vi "Solve General Linear Equations with SVD (CDB).vi"(8 "iteration":i32=2, 9 "relative tolerance":dbl, 10 "Known Vector":cdb[](array[numeric]), 11 "Input Matrix":T1) -> (0 "error":i32, 3 "Solution Vector":cdb[](array[numeric]))   [LabVIEW 2020, in "NI_AALPro.lvlib"]
uses:
  NI_AALPro.lvlib
  ComplexMatrix.ctl
  NI_AALBase.lvlib
  NI_Matrix.lvlib
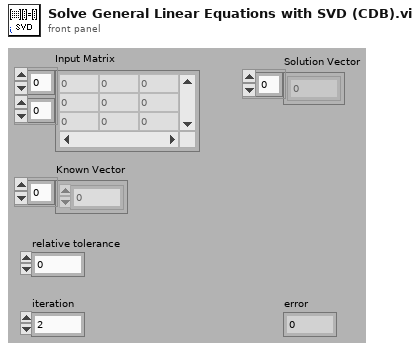
[diagram p1: front panel]
types:
  T1 = typedef "NI_Matrix.lvlib/ComplexMatrix.ctl" = cdb[][]
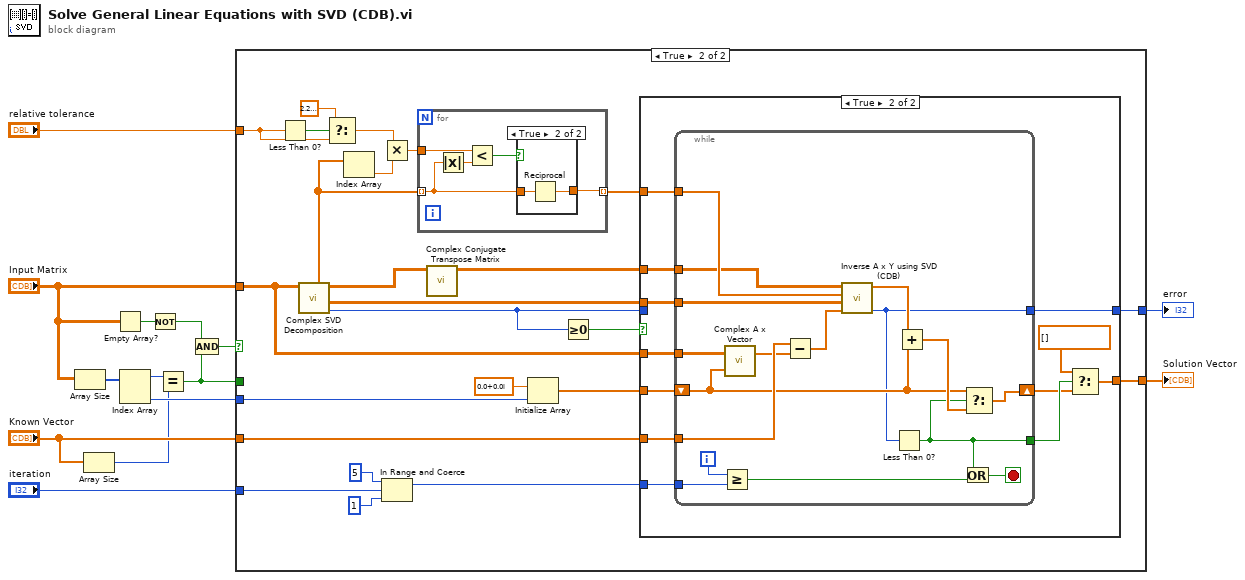
[diagram p0: block diagram]
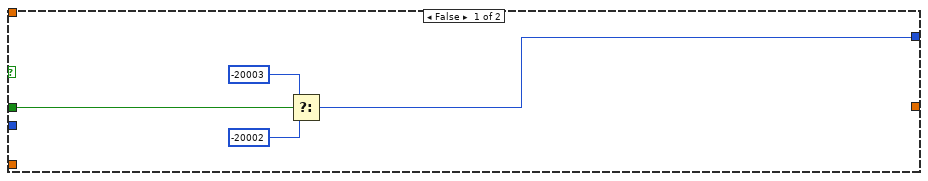
[diagram p2: hidden frame]
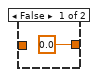
[diagram p4: hidden frame]
diagram:
  n1 = Array Size(array="Input Matrix") -> (size(s)=w12:i32[])
  n2 = Array Size(array="Known Vector") -> (size(s)=w6:i32)
  n3 = Empty Array?(array="Input Matrix") -> (empty?=w4:bool)
  n4 = Index Array(array=w12) -> (element #1=w7:i32, element #2=w9:i32)  [unwired: 2 in]
  n5 = Not(x=w4) -> (.not. x?=w3:bool)
  n6 = Equal?(x=w7, y=w6) -> (x = y?=w1:bool)
  n7 = Compound Arithmetic op=AND(w3, w1) -> (w2:bool)
  n8 = case shown="True" w2 {
    tunnel: "relative tolerance" -> [_ w41]
    tunnel: "iteration" -> [_ w31]
    tunnel: "Input Matrix" -> [_ w19]
    tunnel: [_ w24] -> w11
    tunnel: [w15 w23] -> w10
    tunnel: w9 -> [_ w21]
    tunnel: "Known Vector" -> [_ w20]
    tunnel: w1 -> [w18 _]
    frame False {
      n9 = Select(t=-20003 ("error"), s=w18, f=-20002 ("error")) -> (s? t:f=w15:i32)
    }
    frame True {
      n10 = Less Than 0?(x=w41) -> (x < 0?=w42:bool)
      n11 = call "Complex SVD Decomposition.vi"("A"=w19) -> ("error"=w22:i32, "Matrix V"=w34:T1, "Matrix U"=w35:T1, "Vector S"=w36:dbl[])  [unwired: 6 in, 1 out]
      n12 = Select(t=2.220446049250313e-16, s=w42, f=w41) -> (s? t:f=w39:dbl)
      n13 = Index Array(array=w36) -> (element=w38:dbl)  [unwired: 1 in]
      n14 = Multiply(x=w39, y=w38) -> (x*y=w37:dbl)
      n15 = In Range and Coerce(upper limit=5, x=w31, lower limit=1) -> (coerced(x)=w28:i32)  [unwired: 1 out]
      n16 = for {
        tunnel: w36 -> [w75] mode=indexing
        tunnel: w37 -> [w77]
        tunnel: [w73] -> w27 mode=indexing
        n17 = Absolute Value(x=w75) -> (abs(x)=w76:dbl)
        n18 = Less?(x=w77, y=w76) -> (x < y?=w74:bool)
        n19 = case shown="True" w74 {
          tunnel: w75 -> [_ w80]
          tunnel: [0.0 w79] -> w73
          frame False {
          }
          frame True {
            n20 = Reciprocal(x=w80) -> (1/x=w79:dbl)
          }
        }
      }
      n21 = call "Complex Conjugate Transpose Matrix.vi"("Input Matrix"=w35) -> ("Matrix Conjugate Transpose"=w33:T1)  [unwired: 9 in, 1 out]
      n22 = Initialize Array(cdb 0.0+0.0i ("element"), w21) -> (w25:cdb[])
      n23 = Greater Or Equal To 0?(x=w22) -> (x >= 0?=w32:bool)
      n24 = case shown="True" w32 {
        tunnel: w34 -> [_ w52]
        tunnel: w33 -> [_ w53]
        tunnel: w19 -> [_ w50]
        tunnel: w20 -> [_ w51]
        tunnel: w28 -> [_ w55]
        tunnel: w27 -> [_ w54]
        tunnel: w25 -> [_ w49]
        tunnel: [_ w44] -> w24
        tunnel: [w43 w48] -> w23
        tunnel: w22 -> [w43 _]
        frame False {
        }
        frame True {
          n25 = while {
            tunnel: w55 -> [w64]
            tunnel: w54 -> [w72]
            tunnel: w53 -> [w71]
            tunnel: w52 -> [w70]
            tunnel: w51 -> [w68]
            tunnel: w50 -> [w69]
            shift-right: [w59] -> w46
            shift-left: w49 -> [w58]
            tunnel: [w57] -> w48
            tunnel: [w56] -> w47
            i -> [w65]
            stop <- w62 stop-if-true
            n26 = Greater Or Equal?(x=w65, y=w64) -> (x >= y?=w63:bool)
            n27 = call "Complex A x Vector.vi"("Vector"=w58, "A"=w69) -> ("A x Vector"=w67:cdb[])  [unwired: 1 out]
            n28 = Subtract(x=w68, y=w67) -> (x-y=w66:cdb[])
            n29 = call "Inverse A x Y using SVD (CDB).vi"("Known Vector"=w66, "V"=w70, "1/S"=w72, "U*"=w71) -> ("error"=w57:i32, "Solution Vector"=w61:cdb[])  [unwired: 6 in]
            n30 = Less Than 0?(x=w57) -> (x < 0?=w56:bool)
            n31 = Add(x=w61, y=w58) -> (x+y=w60:cdb[])
            n32 = Or(x=w56, y=w63) -> (x .or. y?=w62:bool)
            n33 = Select(t=w58, s=w56, f=w60) -> (s? t:f=w59:cdb[])
          }
          n34 = Select(t=cdb[] [], s=w47, f=w46) -> (s? t:f=w44:cdb[])
        }
      }
    }
  }
  "Solution Vector" <- w11
  "error" <- w10
